vi "Guardar datos de Amplitud y Tiempo.vi"(0 "path":path, 1 "Hora inicio":string, 2 "Hora fin":string, 3 "Datos experimento":string[][](array[string]), 4 "column headers":string[](array[string])=["Tiempo", "Amplitud"]) -> ()   [LabVIEW 2016]
uses:
  <vilib>/addons/_office/_exclsub.llb/font.ctl
  <vilib>/addons/_office/excel.llb/Excel Easy Table (str).vi
  <vilib>/Utility/NIReport.llb/NI_report.lvclass
  <vilib>/Utility/NIReport.llb/Excel/NI_Excel.lvclass
  <vilib>/addons/_office/NI_ReportGenerationToolkit.lvlib
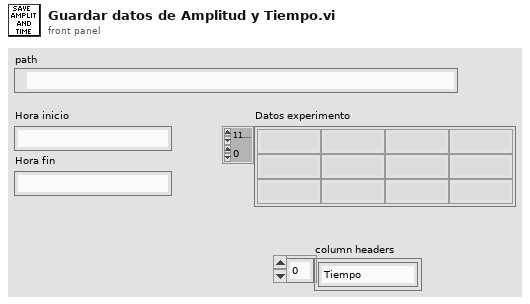
[diagram p1: front panel]
types:
  T1 = typedef "NI_ReportGenerationToolkit.lvlib/font.ctl" = cluster{"font name":string, "font size":dbl, "bold":u16, "italic":u16, "underline":u16, "strike through":u16, "font color":u32}
  T2 = enum16{"Standard Report", "HTML", "Word", "Excel"}
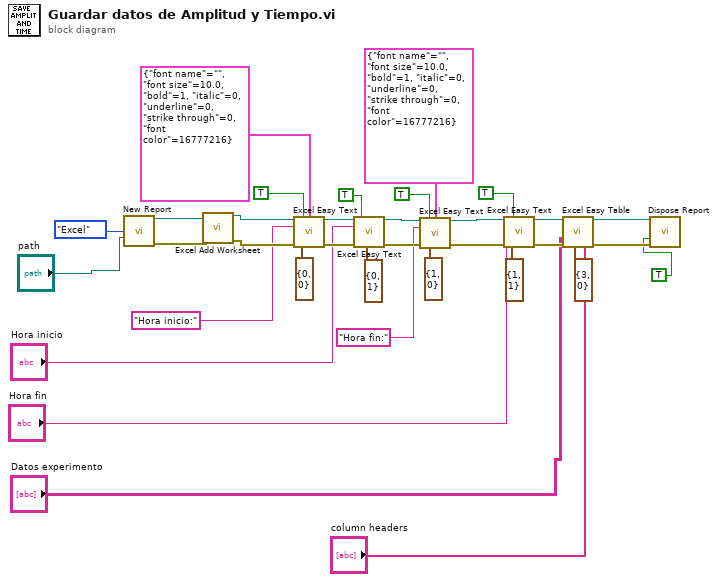
[diagram p0: block diagram]
diagram:
  n1 = call <vilib>:"New Report.vi"("report type"=T2."Excel", "template (empty)"="path") -> ("report out"=w27:refnum<class "NI_report.lvclass">, "error out"=w25:errorcluster)  [unwired: 12 in]
  n2 = call <vilib>:"Excel Add Worksheet.vi"("report in"=w27, "error in (no error)"=w25) -> ("report out"=w26:refnum<class "NI_report.lvclass">, "error out"=w24:errorcluster)  [unwired: 12 in]
  n3 = call <vilib>:"Excel Easy Text.vi"("report in"=w26, "border? (F)"=TRUE, "font"=T1 {"font name"="", "font size"=10.0, "bold"=1, "italic"=0, "underline"=0, "strike through"=0, "font color"=16777216}, "text"="Hora inicio:" ("string"), "start (-1, -1)"=cluster{"row":i32, "column":i32} {"row"=0, "column"=0}, "error in (no error)"=w24) -> ("report out"=w29:refnum<class "NI_report.lvclass">, "error out"=w30:errorcluster)  [unwired: 5 in, 3 out]
  n4 = call <vilib>:"Excel Easy Text.vi"("report in"=w29, "border? (F)"=TRUE, "text"="Hora inicio", "start (-1, -1)"=cluster{"row":i32, "column":i32} {"row"=0, "column"=1}) -> ("report out"=w17:refnum<class "NI_report.lvclass">)  [unwired: 7 in, 4 out]
  n5 = call <vilib>:"Excel Easy Text.vi"("report in"=w17, "border? (F)"=TRUE, "font"=T1 {"font name"="", "font size"=10.0, "bold"=1, "italic"=0, "underline"=0, "strike through"=0, "font color"=16777216}, "text"="Hora fin:" ("string"), "start (-1, -1)"=cluster{"row":i32, "column":i32} {"row"=1, "column"=0}) -> ("report out"=w13:refnum<class "NI_report.lvclass">)  [unwired: 6 in, 4 out]
  n6 = call <vilib>:"Excel Easy Text.vi"("report in"=w13, "border? (F)"=TRUE, "text"="Hora fin", "start (-1, -1)"=cluster{"row":i32, "column":i32} {"row"=1, "column"=1}) -> ("report out"=w5:refnum<class "NI_report.lvclass">)  [unwired: 7 in, 4 out]
  n7 = call-poly <vilib>:"Excel Easy Table.vi"("report in"=w5, "start (0, 0)"=cluster{"row":i32, "column":i32} {"row"=3, "column"=0}, "text data"="Datos experimento", "column headers"="column headers") -> ("report out"=w4:refnum<class "NI_report.lvclass">)  [unwired: 7 in, 4 out]
  n8 = call-dynamic "Dispose Report.vi"("report in"=w4, "save changes? (F)"=TRUE ("close report? (T)"), "error in (no error)"=w30) -> ()  [unwired: 12 in, 1 out]
